vi "Parse Payload.vi"(8 "error in (no error)":errorcluster, 10 "Include Header":bool, 11 "CIFFIFO in":refnum<class "CIF_NIChn_Fifo_U8.lvclass">) -> (0 "error out":errorcluster, 2 "Data":u8[](array[numeric]), 4 "Header out":T1)   [LabVIEW 2021, in "CIF_NIChn_Fifo_U8.lvclass"]
uses:
  CIF_NIChn_Fifo_U8.lvclass
  CIF_NIChn_Fifo_U8.lvclass/CIF_NIChn_Fifo_U8.ctl
  <vilib>/CIF Foundation/CIF Utilities/DataTypes/Unflatten U64.vi
  <vilib>/CIF Foundation/CIF Utilities/DataTypes/Unflatten I64.vi
  ChannelCommon/Utilities/Add Error.vi
  <vilib>/CIF Foundation/CIF Utilities/Errors/Append Error Location.vi
  ChannelCommon/ChannelCommon.lvlib
  ChannelCommon/typedef/FIFO Header.ctl
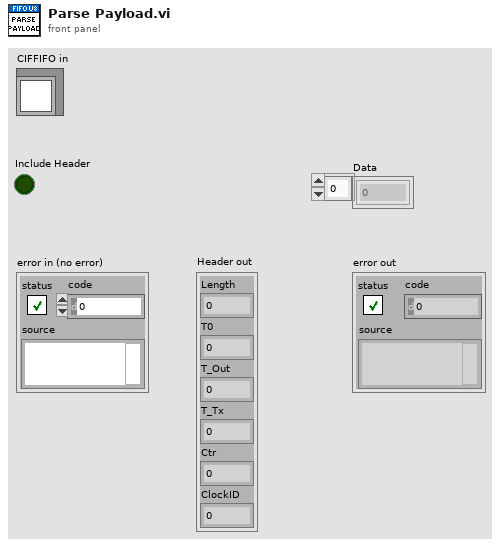
[diagram p1: front panel]
types:
  T1 = typedef "ChannelCommon.lvlib/FIFO Header.ctl" = cluster{"Length":u64, "T0":i64, "T_Out":i64, "T_Tx":i64, "Ctr":u64, "ClockID":u8}
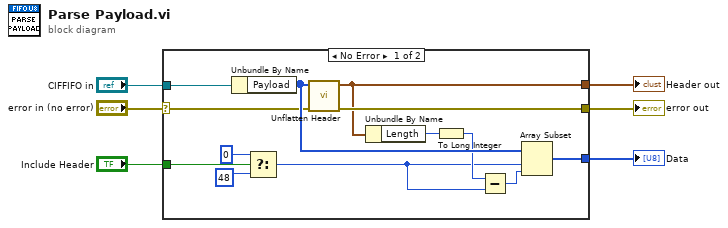
[diagram p0: block diagram]
diagram:
  n1 = case shown="No Error" "error in (no error)" {
    selector: "error in (no error)" -> [w17 w20]
    tunnel: [w16 w20] -> w5
    tunnel: "CIFFIFO in" -> [w18 _]
    tunnel: "Include Header" -> [w12 _]
    tunnel: [w8 _] -> w2
    tunnel: [w7 _] -> w1
    frame No Error {
      n2 = Unbundle By Name(w18) -> ("Payload"=w19:u8[])
      n3 = Select(t=0, s=w12, f=48 ("index")) -> (s? t:f=w9:i32)
      n4 = call "Unflatten Header.vi"("error in (no error)"=w17, "Flattened Data in"=w19) -> ("error out"=w16:errorcluster, "Header out"=w7:T1)  [unwired: 7 in, 1 out]
      n5 = Unbundle By Name(w7) -> ("Length"=w15:u64)
      n6 = To Long Integer(number=w15) -> (32bit integer=w13:i32)
      n7 = Subtract(x=w13, y=w9) -> (x-y=w14:i32)
      n8 = Array Subset(array=w19, index=w9, length=w14) -> (w8:u8[])
    }
    frame Error {
    }
  }
  "error out" <- w5
  "Data" <- w2
  "Header out" <- w1
